vi "MGCC_FntStaMach_Flag manual panel.vi"() -> ()   [LabVIEW 2016]
panel:
  in  "Total MG load < threshold":bool
  in  "Total MG gen < threshold":bool
  in  "PCC_5 IR position":bool
  in  "PCC_4 IR position":bool
  in  "PCC_3 IR position":bool
  in  "PCC_2 IR position":bool
  in  "PCC_1 IR position":bool
  in  "Feeder #5 energized":bool
  in  "Feeder #4 energized":bool
  in  "Feeder #3 energized":bool
  in  "Feeder #2 energized":bool
  in  "Feeder #1 energized":bool
  in  "PCC IR switching off":bool
  in  "Recon. command received":bool
  in  "Blackstart command received":bool
  in  "Islanding command received":bool
  in  "Fault flag":bool
  in  "Abnormal flag":bool
  in  "Ready to run/MG blackout flag":bool
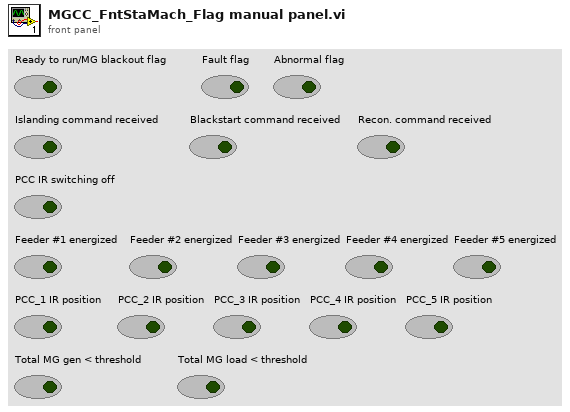
[diagram p1: front panel]
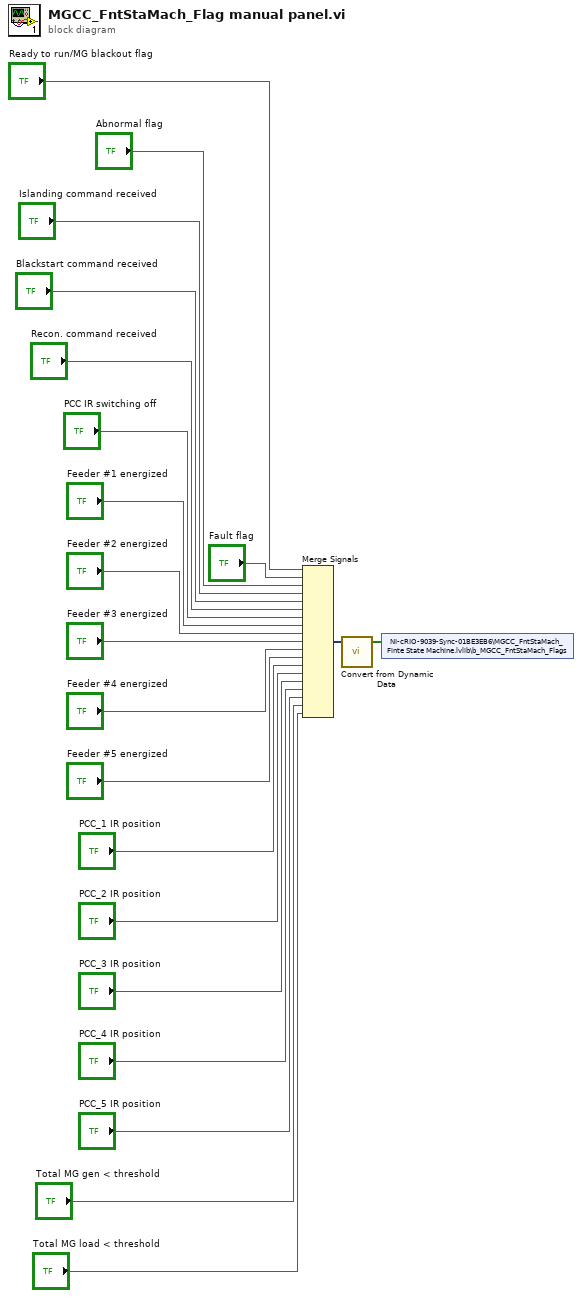
[diagram p0: block diagram]
diagram:
  n1 = Merge Signals("Ready to run/MG blackout flag", "Fault flag", "Abnormal flag", "Islanding command received", "Blackstart command received", "Recon. command received", "PCC IR switching off", "Feeder #1 energized", "Feeder #2 energized", "Feeder #3 energized", "Feeder #4 energized", "Feeder #5 energized", "PCC_1 IR position", "PCC_2 IR position", "PCC_3 IR position", "PCC_4 IR position", "PCC_5 IR position", "Total MG gen < threshold", "Total MG load < threshold") -> (w21:dynamicdata)
  n2 = call "Convert from Dynamic Data"("Dynamic Data Type"=w21) -> ("Array"=w20:bool[])  [unwired: 3 in]
  n3 = shared-variable "NI-cRIO-9039-Sync-01BE3EB6\\MGCC_FntStaMach_Finte State Machine.lvlib\\b_MGCC_FntStaMach_Flags"(w20) -> ()  [unwired: 1 in, 1 out]
